vi "Go.vi"(8 "Timing Data (Go Down and Dispense)":T1(array[cluster]), 9 "Timing Data":dbl[](array[numeric]), 10 "Control In":T2={"I-O.lvclass"=refnum, "Motion.lvclass"=refnum, "Dispenser.lvclass"=refnum}, 11 "CAD Dispense2 in":refnum<class "CAD Dispense2.lvclass">) -> (2 "Control Out":T2, 3 "CAD Dispense2 Out":refnum<class "CAD Dispense2.lvclass">)   [LabVIEW 2016, in "CAD Dispense2.lvclass"]
uses:
  CAD Dispense2.lvclass
  D:/UCSB-Gantry_ms/UCSB-Gantry 0510/V5/Classes/Routine/Dispense/Dispense.lvclass
  Controller/Controllers.ctl
  Controller/I-O/I-O.lvclass
  Controller/Motion/A3200/A3200.lvclass
  Controller/Dispenser/Dispenser.lvclass
  Controller/Motion/Motion.lvclass
  CAD Dispense2.lvclass/CAD Dispense2.ctl
  Dispense.lvclass/Dispense.ctl
  Read Z Height.vi
  Read Z speed.vi
  Controller/Controller.lvclass
panel:
  out "error out":errorcluster
  in  "error in (no error)":errorcluster
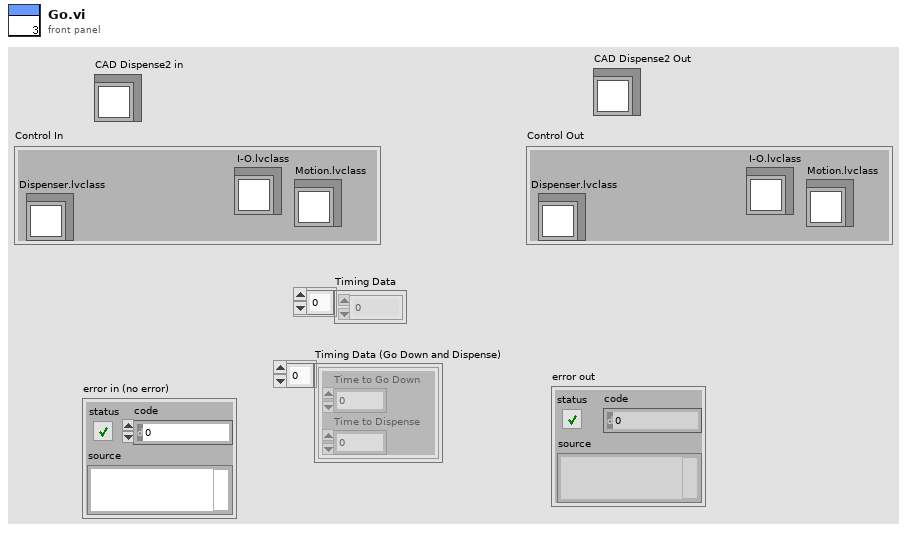
[diagram p1: front panel]
types:
  T1 = cluster{"Time to Go Down":dbl, "Time to Dispense":dbl}[]
  T2 = typedef "Controller.lvclass/Controllers.ctl" = cluster{"I-O.lvclass":refnum<class "I-O.lvclass">, "Motion.lvclass":refnum<class "Motion.lvclass">, "Dispenser.lvclass":refnum<class "Dispenser.lvclass">}
  T3 = cluster{"Endpoints":dbl[][], "Center":dbl[], "Dispense Type":enum16{"N-gon", "Square", "Arc", "Dot", "Line", "Circle"}, "CW/CCW":dbl}[]
  T4 = enum16{"N-gon", "Square", "Arc", "Dot", "Line", "Circle"}
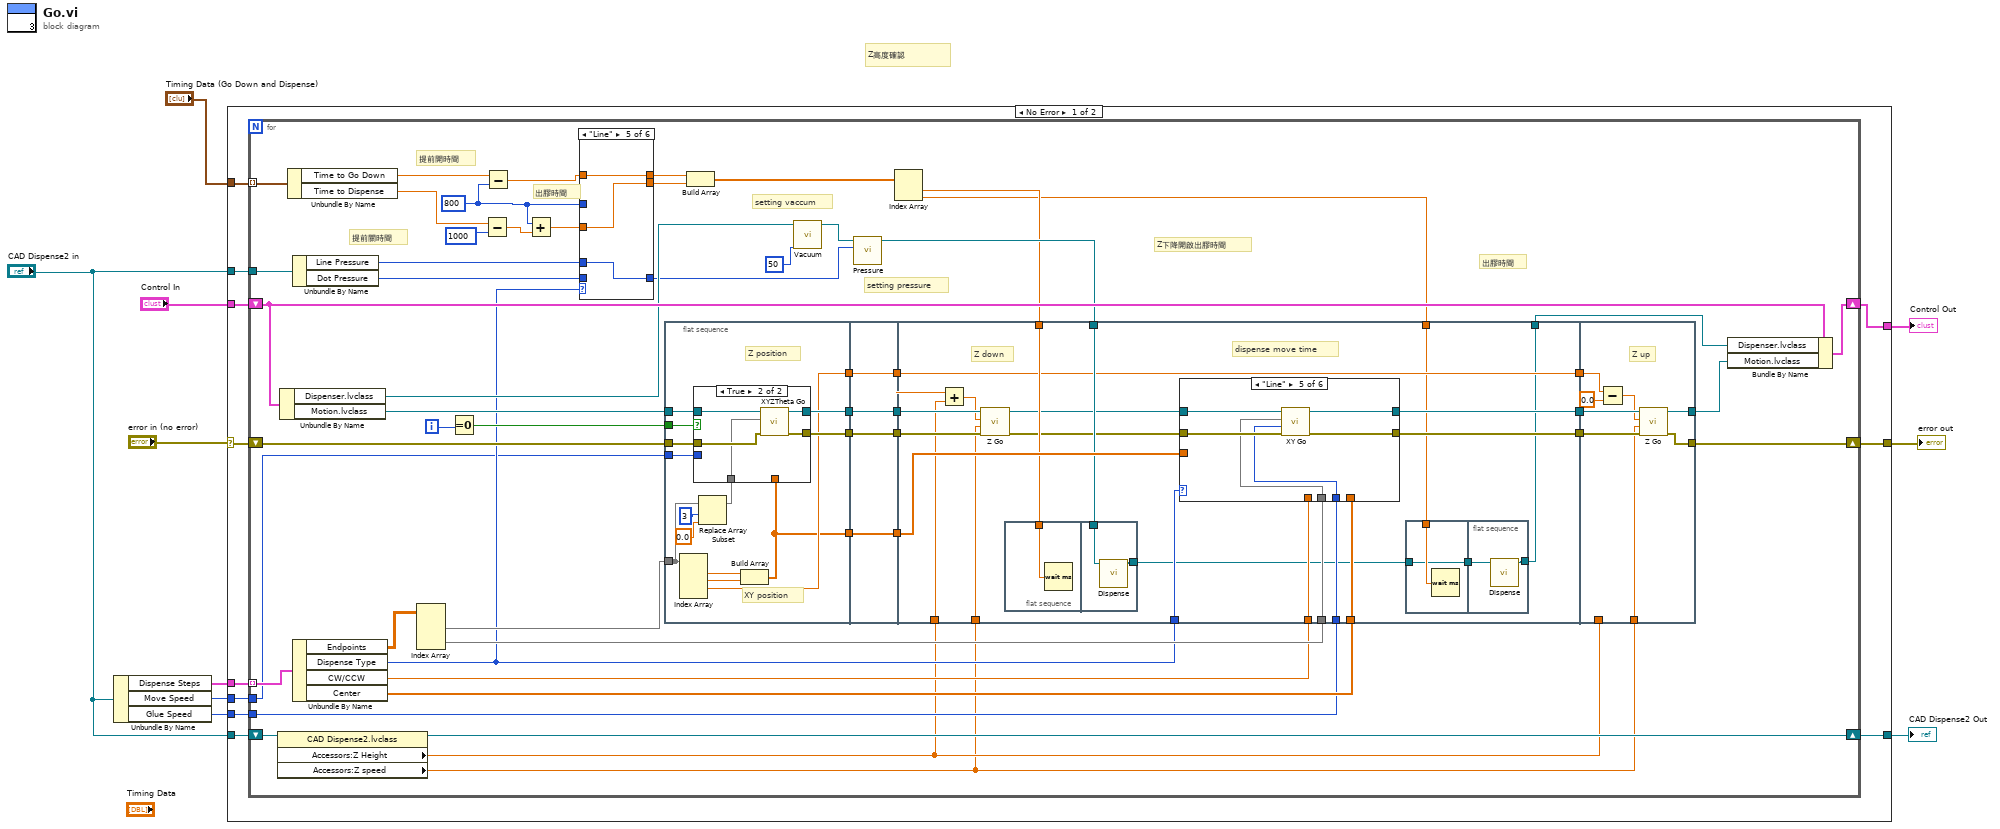
[diagram p0: block diagram]
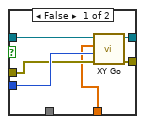
[diagram p2: hidden frame]
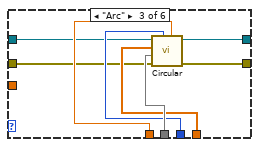
[diagram p5: hidden frame]
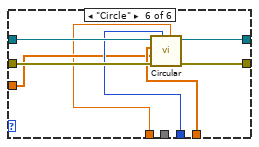
[diagram p7: hidden frame]
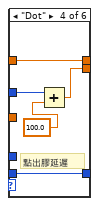
[diagram p11: hidden frame]
diagram:
  # "Z高度確認"
  n1 = Unbundle By Name("CAD Dispense2 in") -> ("Dispense Steps"=w10:T3, "Move Speed"=w7:i32, "Glue Speed"=w6:i32)
  n2 = case shown="No Error" "error in (no error)" {
    selector: "error in (no error)" -> [w13 w192]
    tunnel: w10 -> [w21 _]
    tunnel: "Timing Data (Go Down and Dispense)" -> [w20 _]
    tunnel: "CAD Dispense2 in" -> [w19 w190]
    tunnel: "Control In" -> [w18 w191]
    tunnel: w7 -> [w17 _]
    tunnel: w6 -> [w16 _]
    tunnel: [w15 w190] -> w5
    tunnel: [w14 w191] -> w4
    tunnel: [w12 w192] -> w2
    tunnel: "CAD Dispense2 in" -> [w11 _]
    frame No Error {
      n3 = for {
        tunnel: w21 -> [w75] mode=indexing
        tunnel: w20 -> [w74] mode=indexing
        shift-right: [w72] -> w15
        shift-left: w19 -> [w73]
        shift-right: [w62] -> w14
        shift-left: w18 -> [w61]
        tunnel: w17 -> [w39]
        tunnel: w16 -> [w40]
        shift-right: [w38] -> w12
        shift-left: w13 -> [w63]
        tunnel: w11 -> [w45]
        i -> [w50]
        w22 = 800
        # "出膠時間"
        # "提前關時間"
        # "提前開時間"
        # "Z下降開啟出膠時間"
        # "出膠時間"
        # "setting pressure"
        # "setting vaccum"
        n4 = property class="CAD Dispense2.lvclass"(reference=w73) -> (reference out=w72:refnum<class "CAD Dispense2.lvclass">, "Accessors:Z Height"=w35:dbl, "Accessors:Z speed"=w34:dbl)  [unwired: 1 in, 1 out]
        n5 = Unbundle By Name(w61) -> ("Dispenser.lvclass"=w46:refnum<class "Dispenser.lvclass">, "Motion.lvclass"=w64:refnum<class "Motion.lvclass">)
        n6 = Unbundle By Name(w74) -> ("Time to Go Down"=w28:dbl, "Time to Dispense"=w26:dbl)
        n7 = Unbundle By Name(w45) -> ("Line Pressure"=w43:i64, "Dot Pressure"=w41:i64)
        n8 = Unbundle By Name(w75) -> ("Endpoints"=w55:dbl[][], "Dispense Type"=w44:T4, "CW/CCW"=w51:dbl, "Center"=w52:dbl[])
        n9 = Index Array(array=w55) -> (element #1=w54:dbl[], element #2=w53:dbl[])  [unwired: 4 in]
        n10 = Equal To 0?(x=w50) -> (x = 0?=w49:bool)
        n11 = Subtract(x=w26, y=1000) -> (x-y=w24:dbl)
        n12 = Subtract(x=w28, y=w22) -> (x-y=w27:dbl)
        n13 = Add(x=w22, y=w24) -> (x+y=w23:dbl)
        n14 = case shown="\"Line\"" w44 {
          tunnel: w43 -> [w172 w175 w178 _ w186 w189]
          tunnel: [w172 w175 w178 w183 w186 w189] -> w42
          tunnel: w41 -> [_ _ _ w183 _ _]
          tunnel: w23 -> [w170 w173 w176 _ w185 w187]
          tunnel: w27 -> [w171 w174 w177 w182 w184 w188]
          tunnel: [w170 w173 w176 w179 w185 w187] -> w31
          tunnel: [w171 w174 w177 w182 w184 w188] -> w30
          tunnel: w22 -> [_ _ _ w180 _ _]
          frame "N-gon", Default {
          }
          frame "Square" {
          }
          frame "Arc" {
          }
          frame "Dot" {
            # "點出膠延遲"
            n15 = Add(x=w180, y=100.0) -> (x+y=w179:dbl)
          }
          frame "Line" {
          }
          frame "Circle" {
          }
        }
        n16 = flat-sequence {
          tunnel: w49 -> [w89]
          tunnel: w39 -> [w88]
          tunnel: w64 -> [w87]
          tunnel: [w86] -> w68
          tunnel: [w81] -> w67
          tunnel: w63 -> [w85]
          tunnel: [w84] -> w66
          tunnel: w54 -> [w79]
          tunnel: [w80] -> w65
          tunnel: w68 -> [w102]
          tunnel: w67 -> [w104]
          tunnel: w66 -> [w101]
          tunnel: [w101] -> w59
          tunnel: [w102] -> w58
          tunnel: [w104] -> w57
          tunnel: w65 -> [w103]
          tunnel: [w103] -> w56
          tunnel: w44 -> [w126]
          tunnel: w59 -> [w115]
          tunnel: w58 -> [w114]
          tunnel: [w125] -> w71
          tunnel: [w124] -> w70
          tunnel: w57 -> [w111]
          tunnel: [w111] -> w69
          tunnel: w53 -> [w123]
          tunnel: w40 -> [w122]
          tunnel: w52 -> [w121]
          tunnel: w56 -> [w120]
          tunnel: w51 -> [w119]
          tunnel: w37 -> [w118]
          tunnel: w36 -> [w117]
          tunnel: w35 -> [w112]
          tunnel: w34 -> [w113]
          tunnel: [w109] -> w33
          tunnel: w32 -> [w108]
          tunnel: w71 -> [w169]
          tunnel: w70 -> [w168]
          tunnel: w69 -> [w164]
          tunnel: w34 -> [w167]
          tunnel: [w166] -> w60
          tunnel: [w165] -> w38
          tunnel: w35 -> [_]
          frame #0 {
            # "XY position"
            # "Z position"
            n17 = Index Array(array=w79) -> (element #1=w83:dbl, element #2=w82:dbl, element #3=w81:dbl)  [unwired: 4 in, 1 out]
            n18 = Replace Array Subset(array=w79, new element=0.0 ("new element/subarray"), index=3) -> (w78:dbl[])
            n19 = Build Array(w83, w82) -> (w80:dbl[])
            n20 = case shown="True" w89 {
              tunnel: w88 -> [w95 _]
              tunnel: w87 -> [w94 w100]
              tunnel: [w93 w99] -> w86
              tunnel: w85 -> [w92 w98]
              tunnel: [w91 w97] -> w84
              tunnel: w80 -> [w90 _]
              tunnel: w78 -> [_ w96]
              frame False {
                n21 = call-dynamic "XY Go.vi"("error in (no error)"=w92, "Speed"=w95, "XY"=w90, "Motion in"=w94) -> ("error out"=w91:errorcluster, "Motion out"=w93:refnum<class "Motion.lvclass">)  [unwired: 6 in]
              }
              frame True {
                n22 = call "XYZTheta Go.vi"("error in (no error)"=w98, "XYZTheta In"=w96, "Motion in"=w100) -> ("error out"=w97:errorcluster, "Motion out"=w99:refnum<class "Motion.lvclass">)  [unwired: 6 in, 1 out]
              }
            }
          }
          frame #1 {
          }
          frame #2 {
            # "Z down"
            # "dispense move time"
            n23 = Add(x=w111, y=w112) -> (x+y=w110:dbl)
            n24 = call-dynamic "Z Go.vi"("error in (no error)"=w115, "Speed"=w113, "Position"=w110, "Motion in"=w114) -> ("error out"=w116:errorcluster, "Motion out"=w105:refnum<class "Motion.lvclass">)  [unwired: 6 in]
            n25 = flat-sequence {
              tunnel: w117 -> [w131]
              tunnel: [w133] -> w106
              tunnel: w118 -> [w132]
              frame #0 {
                n26 = Wait (ms)(milliseconds to wait=w131) -> ()  [unwired: 1 out]
              }
              frame #1 {
                n27 = call-dynamic "Dispense.vi"("Dispenser in"=w132) -> ("Dispenser out"=w133:refnum<class "Dispenser.lvclass">)  [unwired: 9 in, 1 out]
              }
            }
            n28 = case shown="\"Line\"" w126 {
              tunnel: w116 -> [w134 w136 w139 w146 w151 w159]
              tunnel: w105 -> [w135 w137 w141 w147 w153 w161]
              tunnel: [w135 w137 w140 w147 w152 w160] -> w125
              tunnel: [w134 w136 w138 w146 w150 w158] -> w124
              tunnel: w123 -> [_ _ w145 _ w149 _]
              tunnel: w122 -> [_ _ w143 _ w148 w157]
              tunnel: w121 -> [_ _ w144 _ _ w156]
              tunnel: w120 -> [_ _ _ _ _ w155]
              tunnel: w119 -> [_ _ w142 _ _ w154]
              frame "N-gon", Default {
              }
              frame "Square" {
              }
              frame "Arc" {
                n29 = call-dynamic "Circular.vi"("Direction"=w142, "Speed"=w143, "error in (no error)"=w139, "XY End"=w145, "XY Center"=w144, "Motion in"=w141) -> ("error out"=w138:errorcluster, "Motion out"=w140:refnum<class "Motion.lvclass">)  [unwired: 4 in]
              }
              frame "Dot" {
              }
              frame "Line" {
                n30 = call-dynamic "XY Go.vi"("error in (no error)"=w151, "Speed"=w148, "XY"=w149, "Motion in"=w153) -> ("error out"=w150:errorcluster, "Motion out"=w152:refnum<class "Motion.lvclass">)  [unwired: 6 in]
              }
              frame "Circle" {
                n31 = call-dynamic "Circular.vi"("Direction"=w154, "Speed"=w157, "error in (no error)"=w159, "XY End"=w155, "XY Center"=w156, "Motion in"=w161) -> ("error out"=w158:errorcluster, "Motion out"=w160:refnum<class "Motion.lvclass">)  [unwired: 4 in]
              }
            }
            n32 = flat-sequence {
              tunnel: w108 -> [w128]
              tunnel: w106 -> [w127]
              tunnel: [w127] -> w107
              tunnel: [w130] -> w109
              tunnel: w107 -> [w129]
              frame #0 {
                n33 = Wait (ms)(milliseconds to wait=w128) -> ()  [unwired: 1 out]
              }
              frame #1 {
                n34 = call-dynamic "Dispense.vi"("Dispenser in"=w129) -> ("Dispenser out"=w130:refnum<class "Dispenser.lvclass">)  [unwired: 9 in, 1 out]
              }
            }
          }
          frame #3 {
            # "Z up"
            n35 = Subtract(x=w164, y=0.0) -> (x-y=w163:dbl)
            n36 = call-dynamic "Z Go.vi"("error in (no error)"=w168, "Speed"=w167, "Position"=w163, "Motion in"=w169) -> ("error out"=w165:errorcluster, "Motion out"=w166:refnum<class "Motion.lvclass">)  [unwired: 6 in]
          }
        }
        n37 = Build Array(w30, w31) -> (w29:dbl[])
        n38 = call-dynamic "Vacuum.vi"("Vacuum Setting (0000)"=i64 50, "Dispenser in"=w46) -> ("Dispenser out"=w47:refnum<class "Dispenser.lvclass">)  [unwired: 8 in, 1 out]
        n39 = call-dynamic "Pressure.vi"("Pressure"=w42, "Dispenser in"=w47) -> ("Dispenser out"=w37:refnum<class "Dispenser.lvclass">)  [unwired: 8 in, 1 out]
        n40 = Index Array(array=w29) -> (element #1=w36:dbl, element #2=w32:dbl)  [unwired: 2 in]
        n41 = Bundle By Name(cluster=w61, "Dispenser.lvclass"=w33, "Motion.lvclass"=w60) -> (w62:T2)
      }
    }
    frame Error {
    }
  }
  "Control Out" <- w4
  "CAD Dispense2 Out" <- w5
  "error out" <- w2
